vi "Print Error.vi"(5 "Custom Device? (T)":bool=TRUE, 7 "error out":errorcluster, 9 "Note (empty)":string, 10 "Your code's public name":string) -> ()   [LabVIEW 2011, in "BK Precision 91xx (GPIB) Custom Device.lvlib"]
doc: "Prints error information out to the console. Provide your code's public name. For example, if your code is about J1939, put that here so the user knows what this printed error information has to do with.\n\nIf this is not a NI VeriStand custom device, write false to the Custom Device? input. This will change the error output and cause this to ignore error -2206.\n\nIf the 'note' field is empty, it is not printed to the console.\n\nExample output 1:\n******J1939 ERROR******\nSource: blah.vi\nCode: 535\n******J1939 ERROR******\n\nExample output 2:\n******XCP and CCP Master CUSTOM DEVICE ERROR******\nSource: blah.vi\nCode: 535\nUser Note: before write\n******XCP and CCP Master CUSTOM DEVICE ERROR******"
uses:
  BK Precision 91xx (GPIB) Custom Device.lvlib
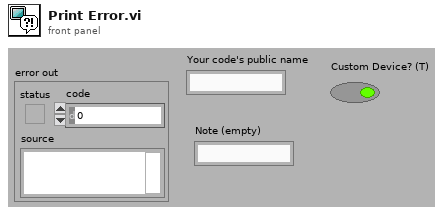
[diagram p1: front panel]
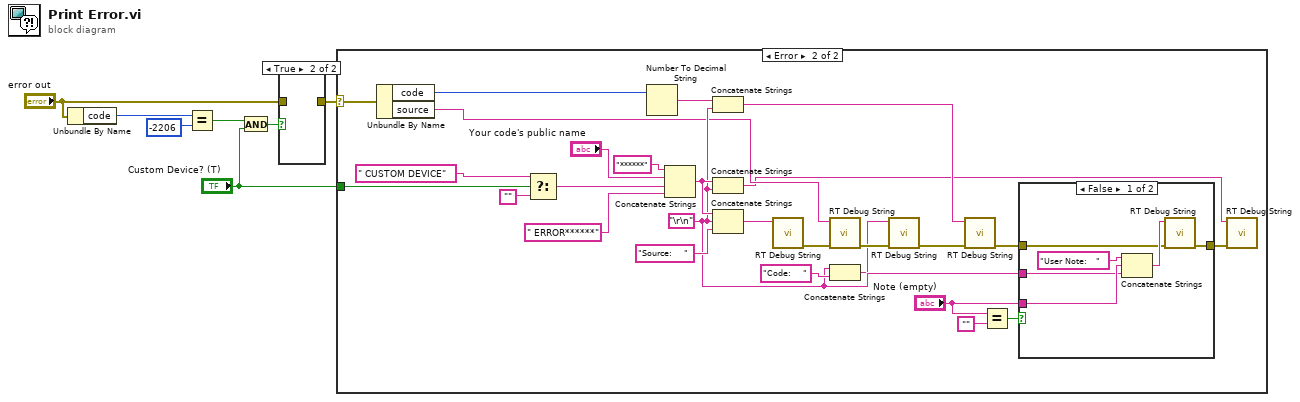
[diagram p0: block diagram]
diagram:
  n1 = Unbundle By Name("error out") -> ("code"=w7:i32)
  n2 = Equal?(x=w7, y=-2206) -> (x = y?=w3:bool)
  n3 = And(x=w3, y="Custom Device? (T)") -> (x .and. y?=w2:bool)
  n4 = case shown="True" w2 {
    tunnel: "error out" -> [w8 _]
    tunnel: [w8 _] -> w4
    frame False {
    }
    frame True {
    }
  }
  n5 = case shown="Error" w4 {
    selector: w4 -> [_ w34]
    tunnel: "Custom Device? (T)" -> [_ w9]
    frame No Error {
    }
    frame Error {
      w19 = "\r\n"
      n6 = Unbundle By Name(w34) -> ("code"=w33:i32, "source"=w17:string)
      n7 = Select(t=" CUSTOM DEVICE" ("String"), s=w9, f="") -> (s? t:f=w10:string)
      n8 = Number To Decimal String(number=w33) -> (decimal integer string=w29:string)  [unwired: 1 in]
      n9 = Concatenate Strings("******" ("String"), "Your code's public name", w10, " ERROR******" ("String")) -> (w23:string)
      n10 = Concatenate Strings(w29, w19) -> (w15:string)
      n11 = Concatenate Strings(w23, w19) -> (w12:string)
      n12 = Concatenate Strings(w23, w19, "Source:    " ("String")) -> (w18:string)
      n13 = call "RT Debug String.vi"("String to write"=w18) -> ("error out"=w35:errorcluster)  [unwired: 10 in]
      n14 = call "RT Debug String.vi"("error in (no error)"=w35, "String to write"=w17) -> ("error out"=w32:errorcluster)  [unwired: 9 in]
      n15 = Concatenate Strings(w19, "Code:    " ("String")) -> (w16:string)
      n16 = call "RT Debug String.vi"("error in (no error)"=w32, "String to write"=w16) -> ("error out"=w28:errorcluster)  [unwired: 9 in]
      n17 = call "RT Debug String.vi"("error in (no error)"=w28, "String to write"=w15) -> ("error out"=w13:errorcluster)  [unwired: 9 in]
      n18 = Equal?(x="Note (empty)", y="") -> (x = y?=w21:bool)
      n19 = case shown="False" w21 {
        tunnel: "Note (empty)" -> [w40 _]
        tunnel: w19 -> [w39 _]
        tunnel: [w37 w42] -> w14
        tunnel: w13 -> [w36 w42]
        frame False {
          n20 = Concatenate Strings("User Note:   " ("string"), w40, w39) -> (w38:string)
          n21 = call "RT Debug String.vi"("error in (no error)"=w36, "String to write"=w38) -> ("error out"=w37:errorcluster)  [unwired: 9 in]
        }
        frame True {
        }
      }
      n22 = call "RT Debug String.vi"("error in (no error)"=w14, "String to write"=w12) -> ()  [unwired: 9 in, 1 out]
    }
  }
